vi "p03.vi"() -> ()   [LabVIEW 2019]
uses:
  <vilib>/Platform/TimedLoop/XDataNode/timing_clust.ctl
  <vilib>/Platform/TimedLoop/XDataNode/nitl_modes.ctl
  <vilib>/Platform/TimedLoop/XDataNode/wakeup.ctl
  <vilib>/DAQmx/read.llb/DAQmx Read (Analog 1D DBL 1Chan NSamp).vi
  <vilib>/Analysis/baseanly.llb/Mean (DBL).vi
  <vilib>/DAQmx/create/channels.llb/DAQmx Create Channel (AI-Voltage-Basic).vi
  <vilib>/DAQmx/configure/timing.llb/DAQmx Timing (Sample Clock).vi
  <vilib>/DAQmx/miscellaneous.llb/DAQmx Fill In Error Info.vi
  <vilib>/Utility/file.llb/Write Delimited Spreadsheet (DBL).vi
  <vilib>/platform/TimedLoop/XDataNode/XDataNode.xnode
  <vilib>/Platform/TimedLoop/XDataNode/XDNodeRunTimeDep.lvlib
  <vilib>/Analysis/NI_AALBase.lvlib
panel:
  in  "Valor Maximo en Celcius":dbl=50.0
  in  "Valor T0":dbl=298.15
  in  "Valor Beta":dbl=4100.0
  in  "Valor Resistencia":dbl=10000.0
  out "Temperatura en K":dbl(graph)
  out "Resistencia en Ohm":dbl(graph)
  out "mean":dbl format="%0.2f"
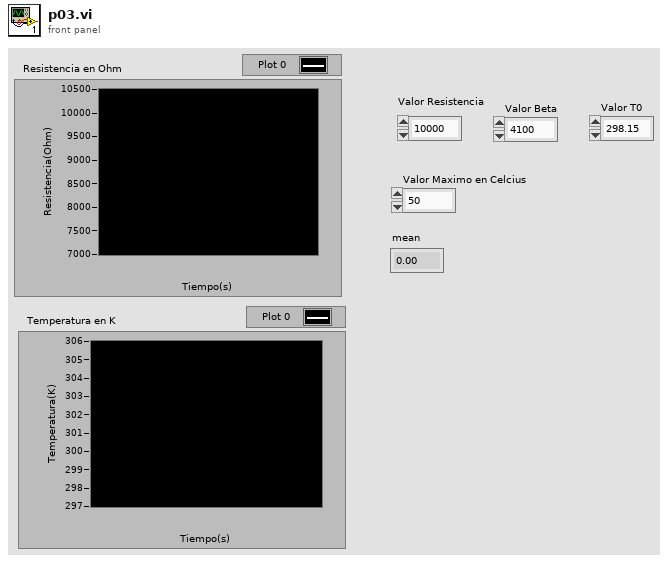
[diagram p1: front panel]
types:
  T1 = typedef "XDNodeRunTimeDep.lvlib/timing_clust.ctl" = cluster{"Expected End [f-1]":u64, "Actual End [f-1]":u64, "Finished Late? [f-1]":bool, "Expected End [i-1]":u64, "Actual End [i-1]":u64, "Finished Late? [i-1]":bool, "Expected Start [i]":u64, "Actual Start [i]":u64, "Expected Start [f]":u64, "Actual Start [f]":u64, "Source Name":string, "Structure Name":string, "Period":i64, "Deadline":i64, "Offset":i64, "Start":i64, "Priority":i32, "Timeout":i32, "Mode":T2, "Wakeup Reason":T3, "Error":errorcluster, "Source Type":string, "Secondary Source Type":string, "Global End Time":u64, "Global Start Time":u64, "Frame Duration":u64, "Iteration Duration":u64, "Assigned CPU":i32, "I/O Scan Engine Mode":u32}
  T2 = typedef "XDNodeRunTimeDep.lvlib/nitl_modes.ctl" = enum32{"No Change", "Process missed periods, maintain original phase", "Discard missed periods, maintain original phase", "Process missed periods, ignore original phase", "Discard missed periods, ignore original phase"}
  T3 = typedef "XDNodeRunTimeDep.lvlib/wakeup.ctl" = enum32{"Normal", "Aborted", "Asynchronous wakeup", "Timing source error", "Timed loop error", "Timeout"}
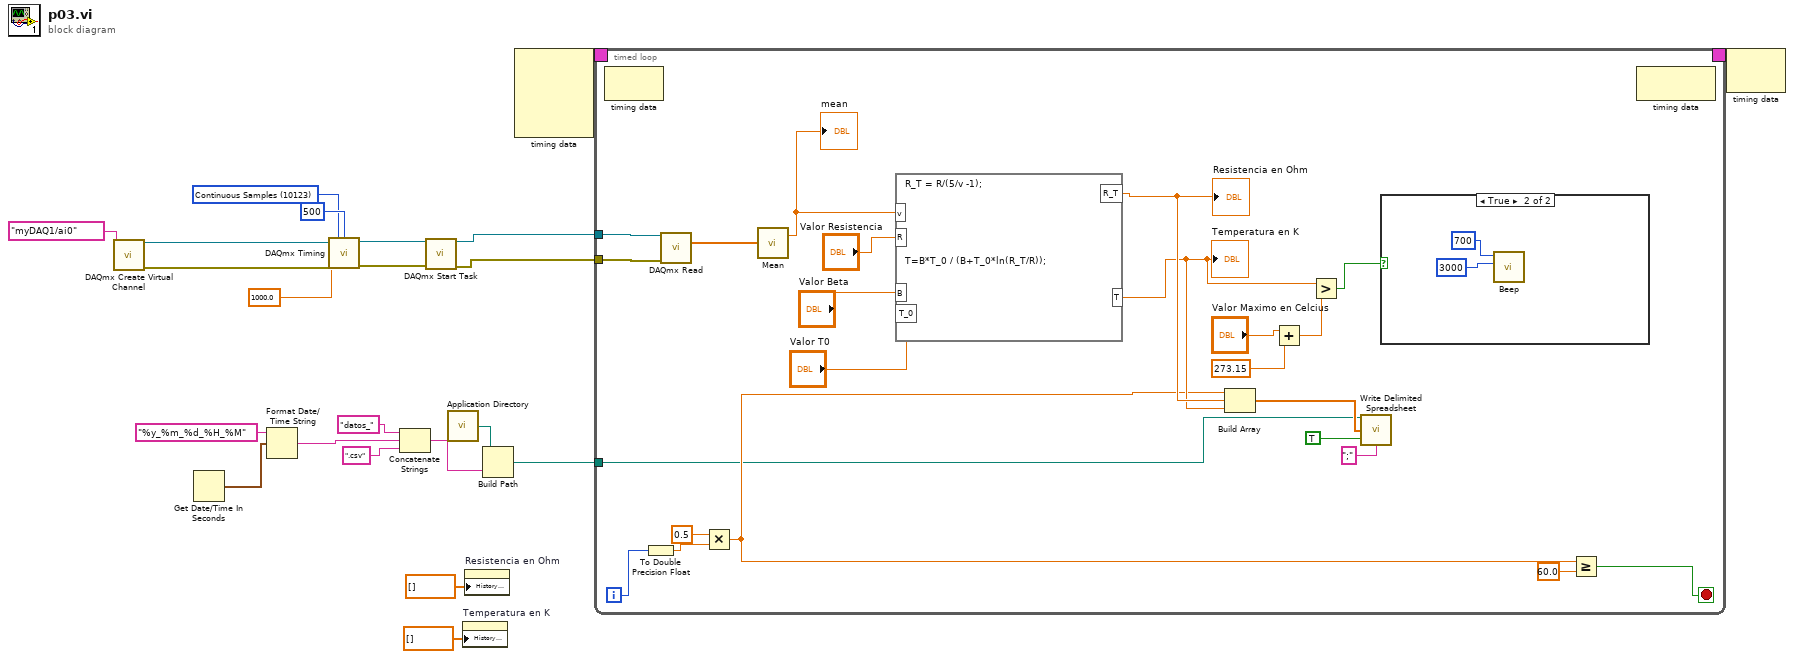
[diagram p0: block diagram]
diagram:
  w12 = 10123 items=["Finite Samples"=10178, "Continuous Samples"=10123, "Hardware Timed Single Point"=12522] ("sample mode")
  n1 = call-poly <vilib>:"DAQmx Create Virtual Channel.vi"("physical channels"=tag "myDAQ1/ai0") -> ("task out"=w22:refnum<k21>, "error out"=w21:errorcluster)  [unwired: 13 in]
  n2 = Get Date/Time In Seconds() -> (seconds since 1Jan1904=w3:timestamp)
  n3 = Format Date/Time String(time format string (%c)="%y_%m_%d_%H_%M", seconds (now)=w3) -> (date/time string=w5:string)  [unwired: 1 in]
  n4 = call-poly <vilib>:"DAQmx Timing.vi"("task/channels in"=w22, "sample mode"=w12, "samples per channel"=500, "rate"=1000.0, "error in"=w21) -> ("task out"=w16:refnum<k21>, "error out"=w15:errorcluster)  [unwired: 9 in]
  n5 = Concatenate Strings("datos_" ("string"), w5, ".csv" ("string")) -> (w8:string)
  n6 = call <vilib>:"DAQmx Start Task.vi"("task/channels in"=w16, "error in"=w15) -> ("task out"=w14:refnum<k21>, "error out"=w13:errorcluster)  [unwired: 12 in]
  n7 = call <vilib>:"Application Directory.vi"() -> ("Application Directory"=w10:path)
  n8 = property on="Temperatura en K" class="WFChart (strict)"("History Data"=dbl[] []) -> ()  [unwired: 2 in, 2 out]
  n9 = property on="Resistencia en Ohm" class="WFChart (strict)"("History Data"=dbl[] []) -> ()  [unwired: 2 in, 2 out]
  n10 = Build Path(base path=w10, name or relative path=w8) -> (appended path=w7:path)
  n11 = node-c288() -> (w18:T1)  [unwired: 4 in]
  n12 = timed-loop {
    timing: w18 -> [_]
    timing-out: [_] -> w17
    tunnel: w14 -> [w45]
    tunnel: w13 -> [w44]
    tunnel: w7 -> [w23]
    i -> [w38]
    stop <- w24 stop-if-true
    n13 = node-c288() -> ()  [unwired: 1 in, 1 out]
    n14 = To Double Precision Float(number=w38) -> (double precision float=w37:dbl)
    n15 = call-poly <vilib>:"DAQmx Read.vi"("task/channels in"=w45, "error in"=w44) -> ("data"=w43:dbl[])  [unwired: 11 in, 2 out]
    n16 = Multiply(x=0.5, y=w37) -> (x*y=w26:dbl)
    n17 = call-poly <vilib>:"Mean.vi"("X"=w43) -> ("mean"=w42:dbl)  [unwired: 1 out]
    "mean" <- w42
    n18 = formula code="R_T = R/(5/v -1);\n\n\n\n\n\n\nT=B*T_0 / (B+T_0*ln(R_T/R));"("v"=w42, "B"="Valor Beta", "T_0"="Valor T0", "R"="Valor Resistencia") -> ("R_T"=w35:dbl, "T"=w30:dbl)
    "Resistencia en Ohm" <- w35
    "Temperatura en K" <- w30
    n19 = Build Array(w26, w35, w30) -> (w34:dbl[])
    n20 = Add(x="Valor Maximo en Celcius", y=273.15) -> (x+y=w27:dbl)
    n21 = Greater?(x=w30, y=w27) -> (0:w31:bool)
    n22 = call-poly <vilib>:"Write Delimited Spreadsheet.vi"("file path (dialog if empty)"=w23, "1D data"=w34, "append to file? (new file:F)"=TRUE, "delimiter (\\t)"=";" ("delimiter (\\t)")) -> ()  [unwired: 10 in, 2 out]
    n23 = case shown="True" w31 {
      frame False {
      }
      frame True {
        n24 = call <vilib>:"Beep.vi"("duration (msec)"=u32 3000, "frequency (Hz)"=u32 700) -> ()  [unwired: 10 in]
      }
    }
    n25 = Greater Or Equal?(x=w26, y=60.0) -> (x >= y?=w24:bool)
    n26 = node-c288() -> ()  [unwired: 1 in, 1 out]
  }
  n27 = node-c288(w17) -> ()  [unwired: 1 out]
